vi "Read Sequential Addresses.vi"(7 "Target IC (1-8)":u8, 8 "error in (no error)":errorcluster, 9 "Addresses to Read":u16 format="%0.0f", 10 "Starting Address":u16 format="%04x", 11 "FPGA Sim in":refnum<class "FPGA Sim.lvclass">) -> (0 "error out":errorcluster, 2 "Data":u16[](array[numeric]) format="%04x")   [LabVIEW 2020, in "Unit Tests.lvlib" / "FPGA Sim.lvclass"]
uses:
  FPGA Sim.lvclass
  FPGA Sim.lvclass/FPGA Sim.ctl
  Dependencies/Virtual Memory Unit/Virtual Memory Unit.lvclass
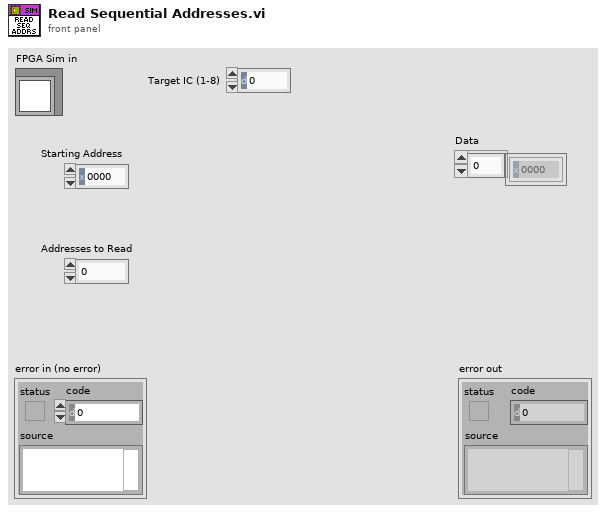
[diagram p1: front panel]
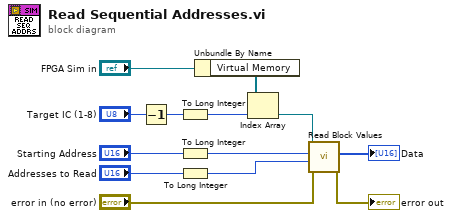
[diagram p0: block diagram]
diagram:
  n1 = Decrement(x="Target IC (1-8)") -> (x-1=w1:u8)
  n2 = To Long Integer(number=w1) -> (32bit integer=w10:i32)
  n3 = To Long Integer(number="Starting Address") -> (32bit integer=w8:i32)
  n4 = To Long Integer(number="Addresses to Read") -> (32bit integer=w3:i32)
  n5 = Unbundle By Name("FPGA Sim in") -> ("Virtual Memory"=w13:refnum<class "Virtual Memory Unit.lvclass">[])
  n6 = Index Array(array=w13, index=w10) -> (element=w9:refnum<class "Virtual Memory Unit.lvclass">)
  n7 = call "Read Block Values.vi"("error in (no error)"="error in (no error)", "Read Length"=w3, "Start Index"=w8, "Virtual Memory Unit in"=w9) -> ("error out"=→"error out":errorcluster, "Read Block"=→"Data":u16[])  [unwired: 6 in]
